vi "Generate Waveform.vi"(0 "signal configuration":refnum<class "SV Sinusoid.lvclass">, 5 "template waveform":waveform(dbl), 9 "samples":i32, 11 "error in (no error)":errorcluster) -> (4 "signal configuration":refnum<class "SV Sinusoid.lvclass">, 6 "sine waveform":waveform(dbl), 10 "samples":i32, 15 "error out":errorcluster)   [LabVIEW 2017, in "SV Sinusoid.lvclass"]
uses:
  <vilib>/addons/_NISVFA/_Generation/Signal Generation/SV Sinusoid/SV Sinusoid.lvclass
  C:/Program Files (x86)/National Instruments/LabVIEW 2017/vi.lib/addons/_NISVFA/_Generation/Signal Generation/SV Signal/SV Signal.lvclass
  C:/Program Files (x86)/National Instruments/LabVIEW 2017/vi.lib/addons/_NISVFA/_Generation/Signal Generation/SV Function/SV Function.lvclass
  <vilib>/addons/_NISVFA/_Generation/Signal Generation/SV Signal/sv_Signal State Attribute.ctl
  <vilib>/addons/_NISVFA/_Generation/Signal Generation/SV Signal/Read Sample Rate.vi
  <vilib>/Analysis/NI_AALBase.lvlib
  <vilib>/addons/_NISVFA/_Generation/Signal Generation/SV Function/SV Function.lvclass
  <vilib>/addons/_NISVFA/_Generation/Signal Generation/SV Signal/SV Signal.lvclass
  <vilib>/measure/NI_MABase.lvlib
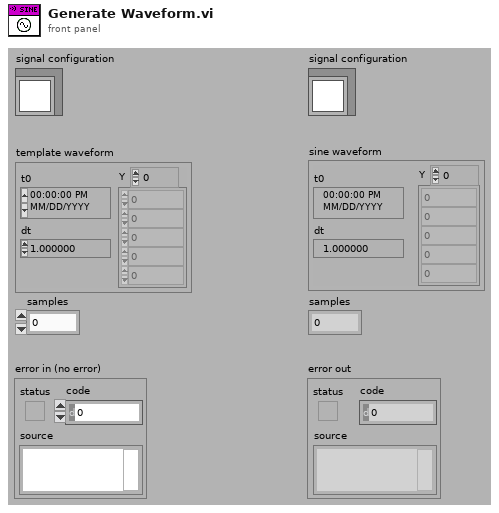
[diagram p1: front panel]
types:
  T1 = typedef "SV Signal.lvclass/sv_Signal State Attribute.ctl" = string
  T2 = typedef "SV Signal.lvclass/sv_System Timing Model.ctl" = i64
  T3 = typedef "SV Signal.lvclass/sv_Generation State.ctl" = enum16{"Idle", "Ramp Up", "Pre-Measurement Settling", "Measurement", "Post-Measurement Settling", "Discrete Sweep Transition", "Ramp Down", "Update"}
  T4 = cluster{"system timing model":T2, "state":cluster{"RESET":bool, "generator timestamp":timestamp, "elapsed seconds":dbl, "elapsed samples":u64, "generation state":T3, "time offset at state":dbl, "samples generated at state":u64, "signal state":variant}, "duration of state":dbl, "samples remaining at state":i32}
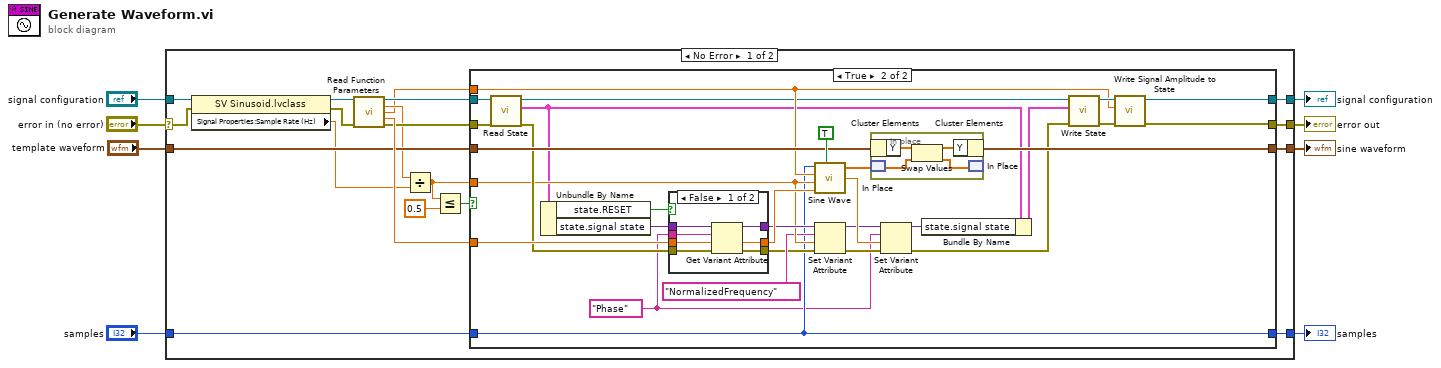
[diagram p0: block diagram]
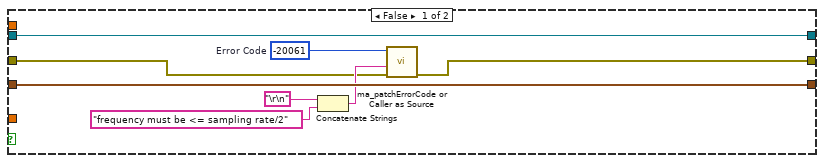
[diagram p2: hidden frame]
diagram:
  n1 = case shown="No Error" "error in (no error)" {
    selector: "error in (no error)" -> [w9 w81]
    tunnel: [w16 w81] -> w7
    tunnel: [w17 w80] -> w5
    tunnel: "signal configuration" -> [w10 w80]
    tunnel: [w27 w79] -> w4
    tunnel: [w14 _] -> w3
    tunnel: "samples" -> [w26 _]
    tunnel: "template waveform" -> [w23 w79]
    frame No Error {
      n2 = property class="SV Sinusoid.lvclass"(reference=w10, error in=w9) -> (reference out=w20:refnum<class "SV Sinusoid.lvclass">, error out=w21:errorcluster, "Signal Properties:Sample Rate (Hz)"=w19:dbl)
      n3 = call <vilib>:"Read Function Parameters.vi"("signal configuration"=w20, "error in (no error)"=w21) -> ("signal configuration"=w25:refnum<class "SV Sinusoid.lvclass">, "frequency_Hz"=w18:dbl, "amplitude"=w15:dbl, "initial_phase_deg"=w24:dbl, "error out"=w22:errorcluster)  [unwired: 8 in, 1 out]
      n4 = Divide(x=w18, y=w19) -> (x/y=w13:dbl)
      n5 = Less Or Equal?(x=w13, y=0.5) -> (x <= y?=w11:bool)
      n6 = case shown="True" w11 {
        tunnel: [w34 w62] -> w27
        tunnel: w26 -> [_ w46]
        tunnel: w25 -> [w35 w45]
        tunnel: w24 -> [_ w61]
        tunnel: w23 -> [w34 w59]
        tunnel: w22 -> [w29 w57]
        tunnel: w13 -> [_ w53]
        tunnel: [w35 w39] -> w17
        tunnel: [w28 w38] -> w16
        tunnel: w15 -> [_ w47]
        tunnel: [_ w46] -> w14
        frame False {
          w30 = -20061  # Error Code
          n7 = Concatenate Strings("\r\n", "frequency must be <= sampling rate/2" ("freq error message")) -> (w33:string)
          n8 = call <vilib>:"ma_patchErrorCode or Caller as Source.vi"("error in (no error)"=w29, "string to append to source"=w33, "error code"=w30) -> ("error out"=w28:errorcluster)  [unwired: 8 in]
        }
        frame True {
          w44 = T1 "Phase" ("name")
          n9 = call <vilib>:"Read State.vi"("signal configuration"=w45) -> ("generator state"=w43:T4, "signal configuration"=w40:refnum<class "SV Sinusoid.lvclass">)  [unwired: 8 in, 1 out]
          n10 = Unbundle By Name(w43) -> ("state.RESET"=w36:bool, "state.signal state"=w41:variant)
          n11 = case shown="False" w36 {
            tunnel: w41 -> [w71 w73]
            tunnel: w61 -> [w70 w74]
            tunnel: [w69 w74] -> w60
            tunnel: [w68 w73] -> w55
            tunnel: w57 -> [w67 w72]
            tunnel: [w66 w72] -> w51
            tunnel: w44 -> [w65 _]
            frame False {
              n12 = Get Variant Attribute(Variant=w71, name=w65, default value (empty Variant)=w70, error in=w67) -> (duplicate Variant=w68:variant, value=w69:dbl, error out=w66:errorcluster)  [unwired: 1 out]
            }
            frame True {
            }
          }
          n13 = call <vilib>:"Sine Wave.vi"("samples"=w46, "amplitude"=w47, "frequency"=w53, "phase in"=w60, "reset phase"=TRUE) -> ("sine wave"=w64:dbl[], "phase out"=w56:dbl)  [unwired: 1 out]
          n14 = Set Variant Attribute(Variant=w55, name=T1 "NormalizedFrequency", value=w53, error in=w51) -> (Variant out=w54:variant, error out=w50:errorcluster)  [unwired: 1 out]
          n15 = in-place {
            n16 = in-place-cluster #1(w59) -> ("Y"=w78:dbl[])
            n17 = in-place-match #2(w64) -> (w76:dbl[])
            n18 = Swap Values(12:w78, 14:w76) -> (1:w77:dbl[], 3:w75:dbl[])  [unwired: 1 in]
            n19 = in-place-cluster #1("Y"=w77) -> (w62:waveform(dbl))
            n20 = in-place-match #2(w75) -> ()  [unwired: 1 out]
          }
          n21 = Set Variant Attribute(Variant=w54, name=w44, value=w56, error in=w50) -> (Variant out=w58:variant, error out=w37:errorcluster)  [unwired: 1 out]
          n22 = Bundle By Name(cluster=w43, "state.signal state"=w58) -> (w42:T4)
          n23 = call <vilib>:"Write State.vi"("error in (no error)"=w37, "generator state"=w42, "signal configuration"=w40) -> ("error out"=w48:errorcluster, "signal configuration"=w49:refnum<class "SV Sinusoid.lvclass">)  [unwired: 7 in]
          n24 = call <vilib>:"Write Signal Amplitude to State.vi"("error in (no error)"=w48, "amplitude"=w47, "SV Signal in"=w49) -> ("error out"=w38:errorcluster, "SV Signal out"=w39:refnum<class "SV Sinusoid.lvclass">)  [unwired: 7 in]
        }
      }
    }
    frame Error {
    }
  }
  "error out" <- w7
  "signal configuration" <- w5
  "sine waveform" <- w4
  "samples" <- w3
